vi "VisualizeNiDaqMx.vi"() -> ()   [LabVIEW 2018, in "Visualization.lvlib" / "VisualizeDigitizer.lvclass"]
doc: "This VI listens for any measurement data associated with the provided PluginName and displays it to the user for analysis. The display is only suitable for data coming from the RoomAlert Plugin."
uses:
  VisualizeDigitizer.lvclass
  <vilib>/event_ctls.llb/usereventprio.ctl
  VisualizeBase/VisualizeBase_class/Requests/clUserEventType.ctl
  SubVI/VisulaizationManagement/PopInOutButton.ctl
  <extravilib>/ChannelInstances/Tag-bool/Write With Abort.vi
  <extravilib>/ChannelInstances/Tag-bool/Read With Abort.vi
  <extravilib>/ChannelInstances/Tag-bool/Instantiate.vi
  <extravilib>/ChannelInstances/Tag-bool/EndpointRead.vi
  <vilib>/Utility/error.llb/Error Cluster From Error Code.vi
  <extravilib>/ChannelInstances/Tag-bool/Endpoint.vi
  <vilib>/ErrorRing/Error Ring.xnode
  <userlib>/NIST/NISTErrorLib/NISTErrorLib.lvlib
  VisualizeBase/VisualizeBase_class/VisualizeBase.lvclass
  <extravilib>/ChannelInstances/Tag-bool.lvlib
  TestClass/Test.lvclass
  Queue/Queue.lvlib
  Digitizer/DigitizerModule/DigitizerModule.lvlib
panel:
  in  "ModuleID":i32
  in  "Log Data":bool
  in  "btnStop":bool
  in  "btnReset":bool
  in  "btnClearTest":bool
  out "Siemens":waveform(dbl)[](graph)=[{"t0"=timestamp(3657200531.6397257 s since 1904-01-01), "dt"=1.0, "Y"=[46.19]}, {"t0"=timestamp(3657200531.6397257 s since 1904-01-01), "dt"=1.0, "Y"=[2.0]}, {"t0"=timestamp(3657200531.6397257 s since 1904-01-01), "dt"=1.0, "Y"=[60.0]}]
  out "ErrorArray":errorcluster[](array[cluster])
  in  "PluginName":string="Sensor.RoomAlert1"
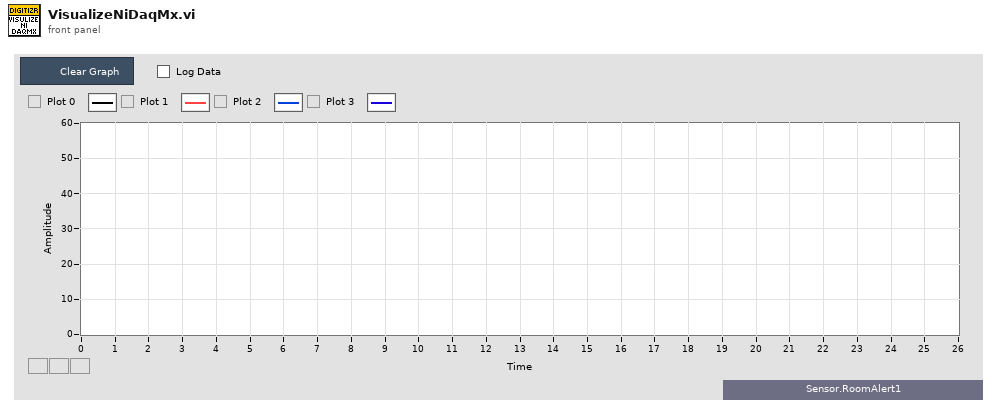
[diagram p1: front panel]
types:
  T1 = enum16{"open", "open or create", "create or replace", "create", "open (read-only)"}
  T2 = typedef "Visualization.lvlib/VisualizeBase.lvclass/clRequestEvents.ctl" = cluster{"StopRequest":refnum<user-event>, "ResetRequest":refnum<user-event>}
  T3 = typedef "DigitizerShared.lvlib/clBroadcastEvents.ctl" = cluster{"DidInit":refnum<user-event>, "StatusUpdate":refnum<user-event>, "ErrorReport":refnum<user-event>, "DidStop":refnum<user-event>, "PathToINI":refnum<user-event>, "Channels":refnum<user-event>, "Acq":refnum<user-event>, "Trigger":refnum<user-event>, "Waveforms":refnum<user-event>}
  T4 = typedef "Visualization.lvlib/VisualizeBase.lvclass/clUserEventType.ctl" = cluster{"BusIndex":i8, "Data":variant}
  T5 = typedef "usereventprio.ctl" = enum32{"high priority", "normal priority"}
  T6 = typedef "Tag-bool.lvlib/))Channel.ctl" = refnum<queue>
  T7 = typedef "PopInOutButton.ctl" = bool
  T8 = typedef "sizeaction.ctl" = enum32{"Minimized", "Maximized", "Resized"}
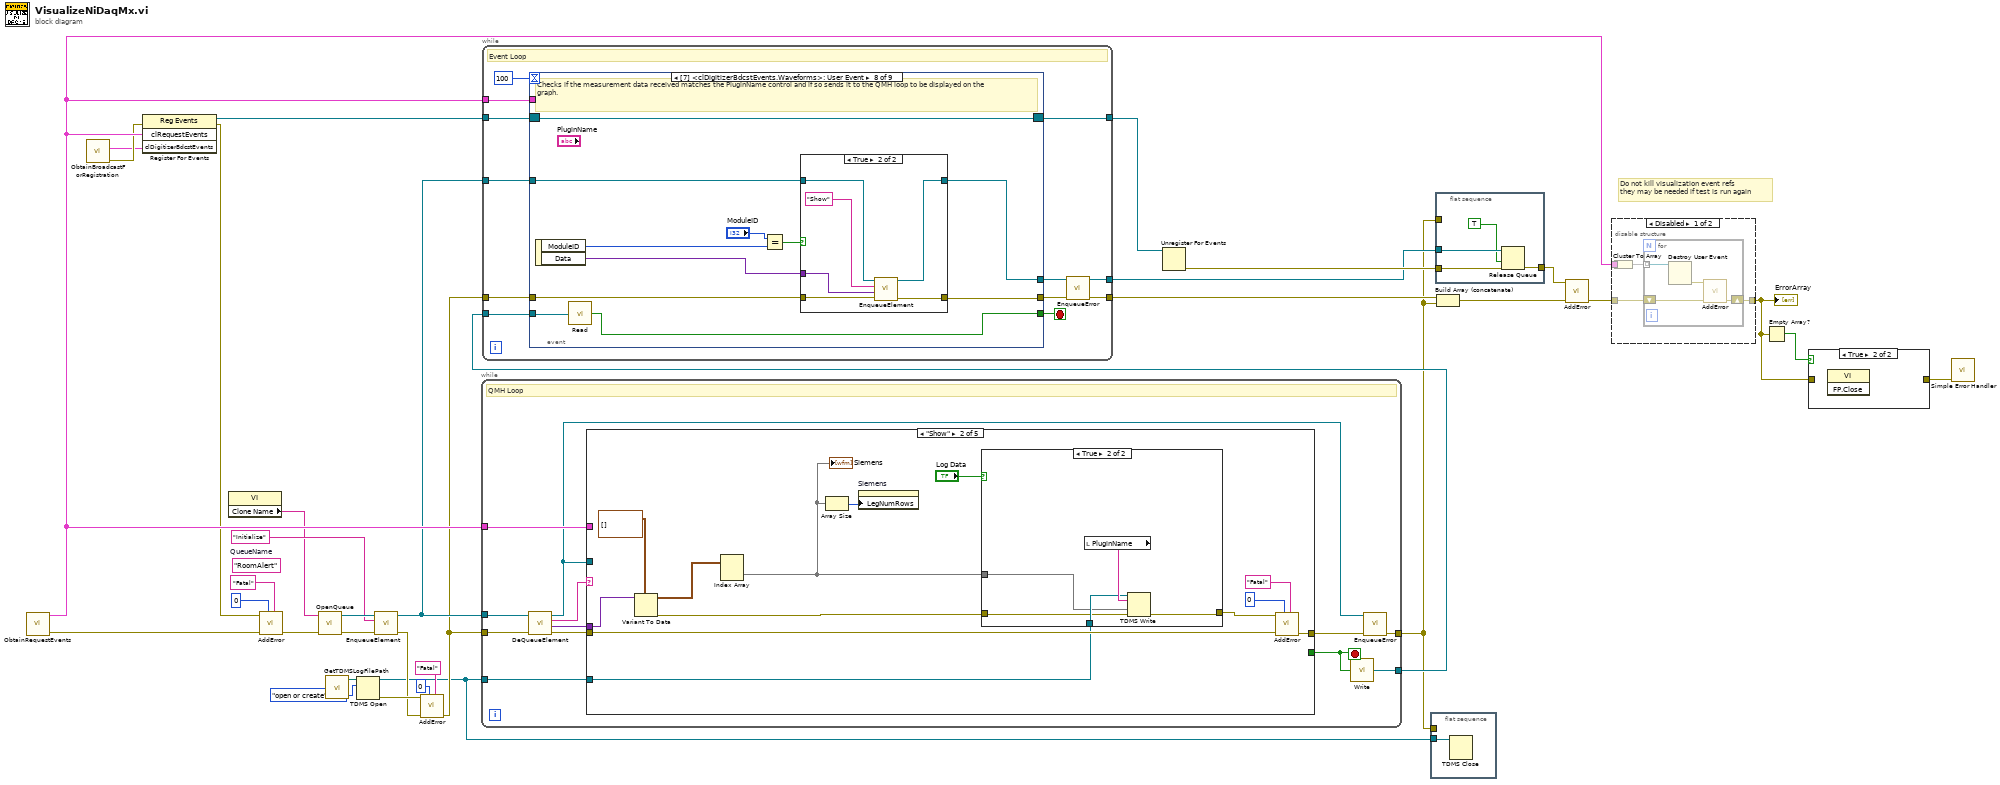
[diagram p0: block diagram]
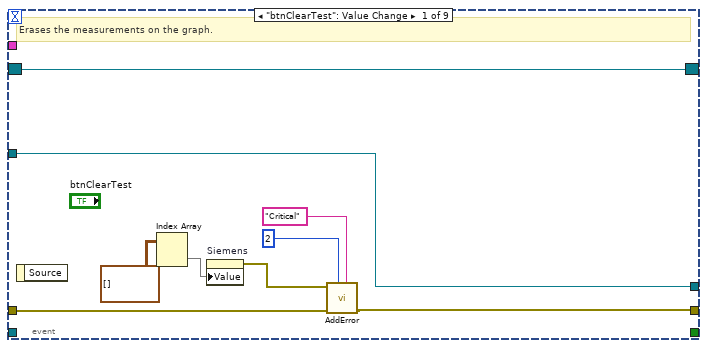
[diagram p3: hidden frame]
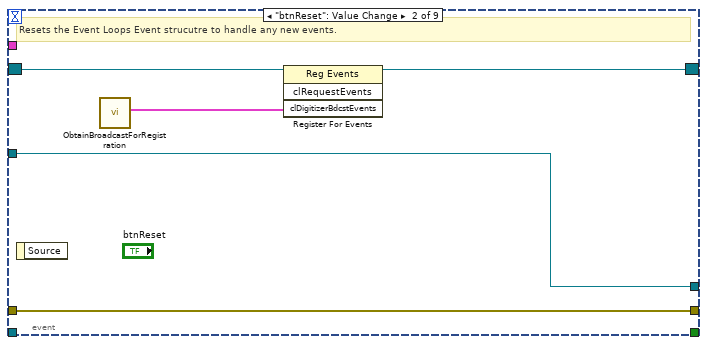
[diagram p4: hidden frame]
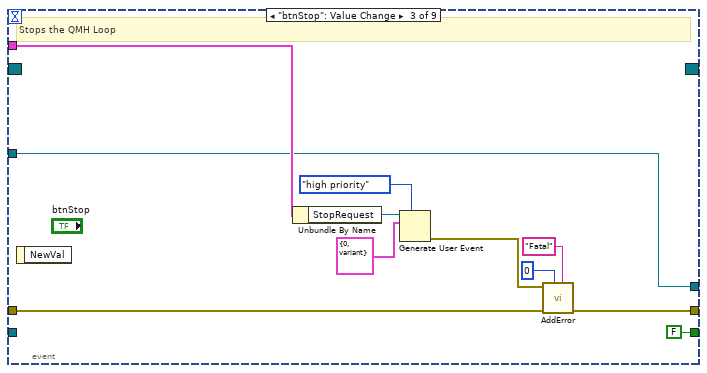
[diagram p5: hidden frame]
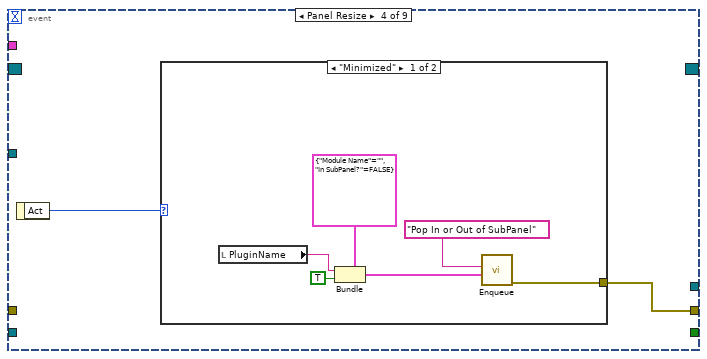
[diagram p6: hidden frame]
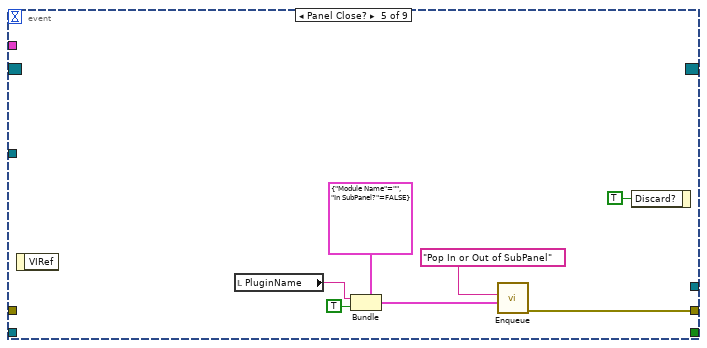
[diagram p8: hidden frame]
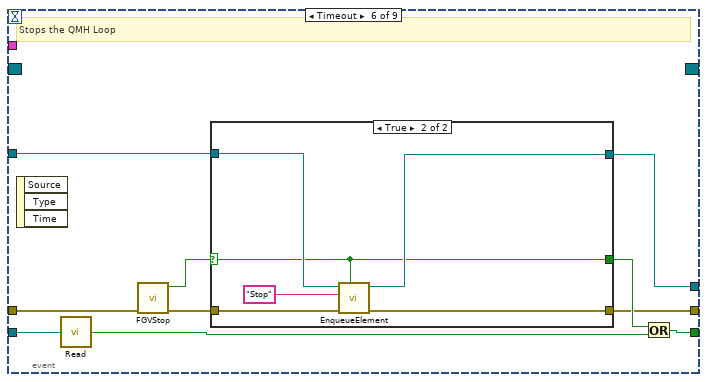
[diagram p9: hidden frame]
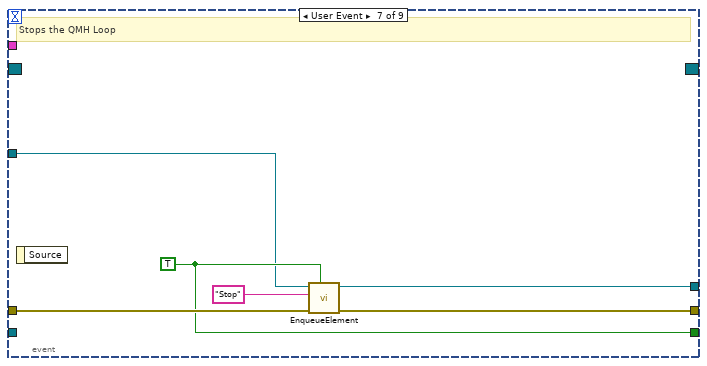
[diagram p11: hidden frame]
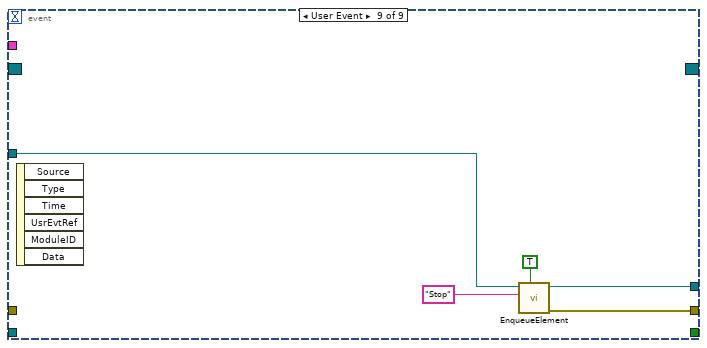
[diagram p13: hidden frame]
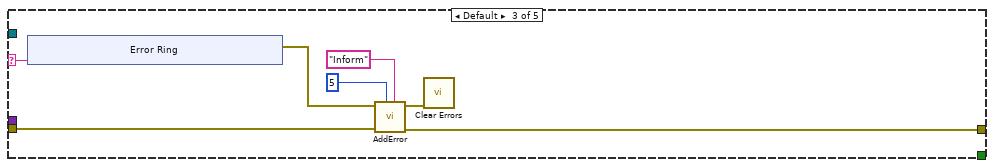
[diagram p16: hidden frame]
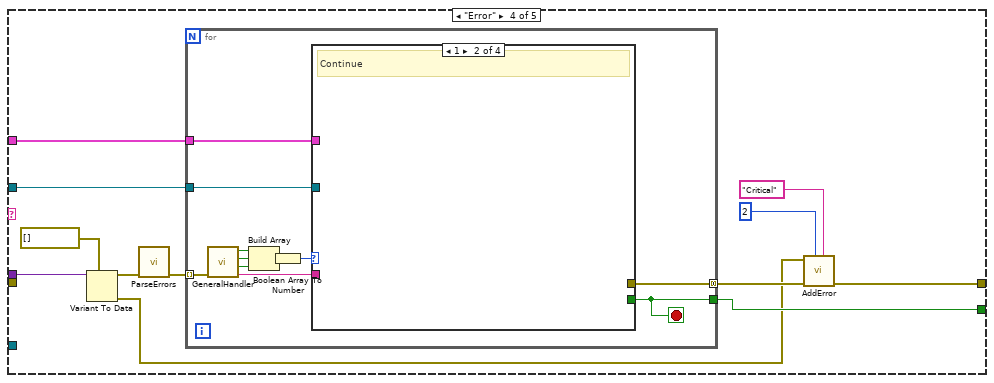
[diagram p17: hidden frame]
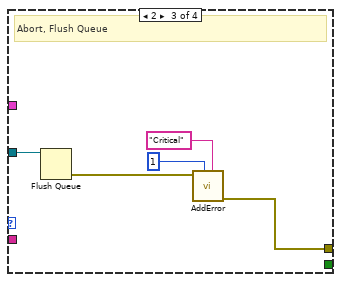
[diagram p19: hidden frame]
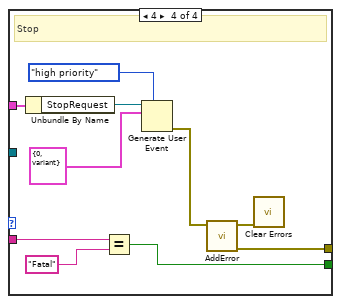
[diagram p20: hidden frame]
diagram:
  (unwired) "RoomAlert"  # QueueName
  # "Do not kill visualization event refs\nthey may be needed if test is run again"
  n1 = call "ObtainRequestEvents.vi"() -> ("Error"=w25:errorcluster[], "clRequestEvents"=w27:T2)  [unwired: 10 in]
  n2 = call "ObtainBroadcastForRegistration.vi"() -> ("error out"=w2:errorcluster, "clDigitizerBdcstEvents"=w1:T3)  [unwired: 10 in]
  n3 = register-events(error in=w2, w27, w1) -> (reference out=w34:refnum<event-registration>, error out=w24:errorcluster)  [unwired: 1 in]
  n4 = property class="VI"() -> ("Clone Name"=w12:string)  [unwired: 2 in, 2 out]
  n5 = call <userlib>:"AddError.vi"("Severity"="Fatal", "Priority"=u8 0, "ErrorArray In"=w25, "error in (no error)"=w24) -> ("ErrorArray Out"=w21:errorcluster[])  [unwired: 6 in, 1 out]
  n6 = call "OpenQueue.vi"("Error Array In"=w21, "QueueName"=w12) -> ("Error Array Out"=w19:errorcluster[], "queue out"=w20:refnum<queue>)  [unwired: 8 in]
  n7 = call "GetTDMSLogFilePath.vi"() -> ("TDMS Log File Path"=w11:path)  [unwired: 11 in]
  n8 = TDMS Open(10:T1."open or create" ("operation (0:open)"), 11:w11) -> (0:w8:errorcluster, 3:w4:refnum<k34>)  [unwired: 5 in]
  n9 = call "EnqueueElement.vi"("Error Array In"=w19, "Message"="Initialize", "queue in"=w20) -> ("Error Array Out"=w7:errorcluster[], "queue out"=w17:refnum<queue>)  [unwired: 7 in]
  n10 = call <userlib>:"AddError.vi"("Severity"="Fatal", "Priority"=u8 0, "ErrorArray In"=w7, "error in (no error)"=w8) -> ("ErrorArray Out"=w6:errorcluster[])  [unwired: 6 in, 1 out]
  n11 = while {
    tunnel: w6 -> [w40]
    tunnel: [w43] -> w3
    tunnel: w17 -> [w39]
    tunnel: w27 -> [w45]
    tunnel: [w36] -> w13
    tunnel: w4 -> [w35]
    stop <- w46 stop-if-true
    # "QMH Loop"
    n12 = call "DeQueueElement.vi"("Error Array In"=w40, "Queue In"=w39) -> ("Error Array Out"=w38:errorcluster[], "Data"=w41:variant, "Message"=w42:string, "Queue Out"=w37:refnum<queue>)  [unwired: 6 in]
    n13 = case shown="\"Show\"" w42 {
      selector: w42 -> [_ _ w73 _ _]
      tunnel: w41 -> [_ w56 _ w92 _]
      tunnel: w38 -> [w47 w59 w71 _ w119]
      tunnel: [w47 w60 w70 w82 w119] -> w44
      tunnel: [_ _ _ w88 TRUE] -> w46
      tunnel: w45 -> [_ _ _ w87 _]
      tunnel: w37 -> [_ _ _ w86 _]
      tunnel: w35 -> [_ w52 _ _ _]
      frame "Initialize" {
      }
      frame "Show" {
        n14 = Variant To Data(type=waveform(dbl)[][] [] ("data"), Variant=w56) -> (data=w49:waveform(dbl)[][], error out=w55:errorcluster)  [unwired: 1 in]
        n15 = Index Array(array=w49) -> (element=w48:waveform(dbl)[])  [unwired: 2 in]
        "Siemens" <- w48
        n16 = Array Size(array=w48) -> (size(s)=w51:i32)
        n17 = property on="Siemens" class="WFGraph (strict)"("LegNumRows"=w51) -> ()  [unwired: 2 in, 2 out]
        n18 = case shown="True" "Log Data" {
          tunnel: w55 -> [w61 w62]
          tunnel: [w61 w66] -> w54
          tunnel: w52 -> [_ w64]
          tunnel: w48 -> [_ w63]
          frame False {
          }
          frame True {
            n19 = local read "PluginName"() -> (w65:string)
            n20 = TDMS Write(0:w64, 5:w65, 9:w63, 11:w62) -> (15:w66:errorcluster)  [unwired: 2 in, 3 out]
          }
        }
        n21 = call <userlib>:"AddError.vi"("Severity"="Fatal" ("String"), "Priority"=u8 0, "ErrorArray In"=w59, "error in (no error)"=w54) -> ("ErrorArray Out"=w60:errorcluster[])  [unwired: 6 in, 1 out]
      }
      frame Default {
        n22 = xnode "Error Ring"("parameter 0"=w73) -> ("error out"=w72:errorcluster)
        n23 = call <userlib>:"AddError.vi"("Severity"="Inform" ("String"), "Priority"=u8 5, "ErrorArray In"=w71, "error in (no error)"=w72) -> ("ErrorArray Out"=w70:errorcluster[], "error out"=w69:errorcluster)  [unwired: 6 in]
        n24 = call <vilib>:"Clear Errors.vi"("error in (no error)"=w69) -> ()  [unwired: 5 in, 2 out]
      }
      frame "Error" {
        n25 = Variant To Data(type=errorcluster[] [], Variant=w92) -> (data=w90:errorcluster[], error out=w81:errorcluster)  [unwired: 1 in]
        n26 = call <userlib>:"ParseErrors.vi"("ErrorArray"=w90) -> ("ErrorArray"=w89:errorcluster[])  [unwired: 8 in, 2 out]
        n27 = for {
          tunnel: w89 -> [w103] mode=indexing
          tunnel: [w97] -> w83 mode=concatenating
          tunnel: [w95] -> w88
          tunnel: w87 -> [w94]
          tunnel: w86 -> [w93]
          stop <- w95 stop-if-true
          n28 = call <userlib>:"GeneralHandler.vi"("error in (no error)"=w103) -> ("Severity"=w96:string, "Stop"=w100:bool, "Abort"=w101:bool, "Continue"=w102:bool)  [unwired: 6 in, 1 out]
          n29 = Build Array(w102, w101, w100) -> (w99:bool[])
          n30 = Boolean Array To Number(Boolean array=w99) -> (number=w98:u32)
          n31 = case shown="1" w98 {
            tunnel: [_ _ w108 w117] -> w97
            tunnel: w96 -> [_ _ _ w110]
            tunnel: [_ _ _ w112] -> w95
            tunnel: w94 -> [_ _ _ w111]
            tunnel: w93 -> [_ _ w104 _]
            frame 0, Default {
              # "No Dialog"
            }
            frame 1 {
              # "Continue"
            }
            frame 2 {
              # "Abort, Flush Queue"
              n32 = Flush Queue(queue=w104) -> (error out=w107:errorcluster)  [unwired: 1 in, 2 out]
              n33 = call <userlib>:"AddError.vi"("Severity"="Critical" ("String"), "Priority"=u8 1, "error in (no error)"=w107) -> ("ErrorArray Out"=w108:errorcluster[])  [unwired: 7 in, 1 out]
            }
            frame 4 {
              # "Stop"
              n34 = Unbundle By Name(w111) -> ("StopRequest"=w118:refnum<user-event>)
              n35 = Equal?(x=w110, y="Fatal" ("x")) -> (x = y?=w112:bool)
              n36 = Generate User Event(priority (normal)=usereventprio."high priority", user event=w118, event data cluster=T4 {"BusIndex"=0, "Data"=variant} ("event data")) -> (error out=w116:errorcluster)  [unwired: 1 in, 1 out]
              n37 = call <userlib>:"AddError.vi"("error in (no error)"=w116) -> ("ErrorArray Out"=w117:errorcluster[], "error out"=w113:errorcluster)  [unwired: 9 in]
              n38 = call <vilib>:"Clear Errors.vi"("error in (no error)"=w113) -> ()  [unwired: 5 in, 2 out]
            }
          }
        }
        n39 = call <userlib>:"AddError.vi"("Severity"="Critical", "Priority"=u8 2, "ErrorArray In"=w83, "error in (no error)"=w81) -> ("ErrorArray Out"=w82:errorcluster[])  [unwired: 6 in, 1 out]
      }
      frame "Stop" {
      }
    }
    n40 = call <extravilib>:"Write.vi"("element"=w46) -> ("channel"=w36:T6)  [unwired: 1 out]
    n41 = call "EnqueueError.vi"("Error Array In"=w44, "Queue in"=w37) -> ("Error Array Out"=w43:errorcluster[])  [unwired: 8 in, 1 out]
  }
  n42 = while {
    tunnel: w34 -> [w132]
    tunnel: [w126] -> w32
    tunnel: [w130] -> w33
    tunnel: w27 -> [w129]
    tunnel: w6 -> [w128]
    tunnel: w17 -> [w127]
    tunnel: [w123] -> w16
    tunnel: w13 -> [w121]
    stop <- w131 stop-if-true
    # "Event Loop"
    n43 = event shown="[7] <clDigitizerBdcstEvents.Waveforms>: User Event" {
      selector: w132 -> [w136 w146 _ _ _ _ _ w204 _]
      dyn-events: [w136 w145 _ _ _ _ _ w204 _] -> w130
      timeout: 100 -> [_ _ _ _ _ _ _ _ _]
      tunnel: [_ _ FALSE ("Priority? (F)") _ _ w173 w194 w201 _] -> w131
      tunnel: [w138 w144 w150 w158 w172 w175 w196 w206 w219] -> w125
      tunnel: w129 -> [_ _ w149 _ _ _ _ _ _]
      tunnel: w128 -> [w139 w144 w157 _ _ w178 w197 w207 _]
      tunnel: w127 -> [w135 w143 w147 _ _ w177 w192 w208 w217]
      tunnel: [w135 w143 w147 _ _ w176 w195 w205 w218] -> w124
      tunnel: w121 -> [_ _ _ _ _ w182 _ w202 _]
      event "btnClearTest": Value Change {
        # "Erases the measurements on the graph."
        n44 = event-data() -> ()  [unwired: 1 in, 1 out]
        n45 = Index Array(array=waveform(dbl)[][] [] ("History Data")) -> (element=w133:waveform(dbl)[])  [unwired: 2 in]
        n46 = property on="Siemens" class="WFGraph (strict)"("Value"=w133) -> (error out=w137:errorcluster)  [unwired: 2 in, 1 out]
        n47 = call <userlib>:"AddError.vi"("Severity"="Critical", "Priority"=u8 2, "ErrorArray In"=w139, "error in (no error)"=w137) -> ("ErrorArray Out"=w138:errorcluster[])  [unwired: 6 in, 1 out]
      }
      event "btnReset": Value Change {
        # "Resets the Event Loops Event strucutre to handle any new events."
        n48 = event-data() -> ()  [unwired: 1 in, 1 out]
        n49 = call "ObtainBroadcastForRegistration.vi"() -> ("clDigitizerBdcstEvents"=w142:T3)  [unwired: 10 in, 1 out]
        n50 = register-events(reference=w146, w142) -> (reference out=w145:refnum<event-registration>)  [unwired: 2 in, 1 out]
      }
      event "btnStop": Value Change {
        # "Stops the QMH Loop"
        n51 = event-data() -> ()  [unwired: 1 in, 1 out]
        n52 = Unbundle By Name(w149) -> ("StopRequest"=w155:refnum<user-event>)
        n53 = Generate User Event(priority (normal)=usereventprio."high priority", user event=w155, event data cluster=T4 {"BusIndex"=0, "Data"=variant} ("event data")) -> (error out=w156:errorcluster)  [unwired: 1 in, 1 out]
        n54 = call <userlib>:"AddError.vi"("Severity"="Fatal" ("String"), "Priority"=u8 0, "ErrorArray In"=w157, "error in (no error)"=w156) -> ("ErrorArray Out"=w150:errorcluster[])  [unwired: 6 in, 1 out]
      }
      event Panel Resize {
        n55 = event-data() -> ("Act"=w159:T8)  [unwired: 1 in]
        n56 = case shown="\"Minimized\"" w159 {
          tunnel: [w160 _] -> w158
          frame "Minimized" {
            n57 = local read "PluginName"() -> (w162:string)
            n58 = Bundle(cluster=cluster{"Module Name":string, "In SubPanel?":T7} {"Module Name"="", "In SubPanel?"=FALSE} ("output cluster"), "Module Name"=w162, "In SubPanel?"=T7 TRUE) -> (w164:cluster{"Module Name":string, "In SubPanel?":T7})
            n59 = call "Enqueue.vi"("Message Data"=w164, "Message"="Pop In or Out of SubPanel") -> ("ErrorArray"=w160:errorcluster[])  [unwired: 9 in]
          }
          frame "Maximized", Default {
          }
        }
      }
      event Panel Close? {
        n60 = event-data() -> ()  [unwired: 1 in, 1 out]
        n61 = local read "PluginName"() -> (w168:string)
        n62 = Bundle(cluster=cluster{"Module Name":string, "In SubPanel?":T7} {"Module Name"="", "In SubPanel?"=FALSE} ("output cluster"), "Module Name"=w168, "In SubPanel?"=T7 TRUE) -> (w170:cluster{"Module Name":string, "In SubPanel?":T7})
        n63 = call "Enqueue.vi"("Message Data"=w170, "Message"="Pop In or Out of SubPanel") -> ("ErrorArray"=w172:errorcluster[])  [unwired: 9 in]
        n64 = event-data("Discard?"=TRUE) -> ()  [unwired: 1 in, 1 out]
      }
      event Timeout {
        # "Stops the QMH Loop"
        n65 = event-data() -> ()  [unwired: 1 in, 3 out]
        n66 = call <extravilib>:"Read.vi"("channel"=w182) -> ("element"=w174:bool)  [unwired: 1 in, 1 out]
        n67 = call "FGVStop.vi"("Error In"=w178) -> ("Error Out"=w180:errorcluster[], "Value"=w181:bool)  [unwired: 9 in]
        n68 = case shown="True" w181 {
          selector: w181 -> [w183 w186]
          tunnel: [w185 w189] -> w175
          tunnel: w180 -> [w185 w190]
          tunnel: w177 -> [w184 w188]
          tunnel: [w184 w187] -> w176
          tunnel: [w183 w186] -> w179
          frame False {
          }
          frame True {
            n69 = call "EnqueueElement.vi"("Priority? (F)"=w186, "Error Array In"=w190, "Message"="Stop", "queue in"=w188) -> ("Error Array Out"=w189:errorcluster[], "queue out"=w187:refnum<queue>)  [unwired: 6 in]
          }
        }
        n70 = Or(x=w179, y=w174) -> (x .or. y?=w173:bool)
      }
      event User Event {
        w194 = TRUE ("Priority? (F)")
        # "Stops the QMH Loop"
        n71 = event-data() -> ()  [unwired: 1 in, 1 out]
        n72 = call "EnqueueElement.vi"("Priority? (F)"=w194, "Error Array In"=w197, "Message"="Stop", "queue in"=w192) -> ("Error Array Out"=w196:errorcluster[], "queue out"=w195:refnum<queue>)  [unwired: 6 in]
      }
      event User Event {
        # "Checks if the measurement data received matches the PluginName control and if so sends it to the QMH loop to be displayed on the graph."
        n73 = event-data() -> ("ModuleID"=w199:i32, "Data"=w200:variant)  [unwired: 1 in]
        n74 = call <extravilib>:"Read.vi"("channel"=w202) -> ("element"=w201:bool)  [unwired: 1 in, 1 out]
        n75 = Equal?(x="ModuleID", y=w199) -> (x = y?=w203:bool)
        n76 = case shown="True" w203 {
          tunnel: [w209 w215] -> w206
          tunnel: w208 -> [w210 w214]
          tunnel: w207 -> [w209 w216]
          tunnel: [w210 w213] -> w205
          tunnel: w200 -> [_ w211]
          frame False {
          }
          frame True {
            n77 = call "EnqueueElement.vi"("Error Array In"=w216, "Data"=w211, "Message"="Show", "queue in"=w214) -> ("Error Array Out"=w215:errorcluster[], "queue out"=w213:refnum<queue>)  [unwired: 6 in]
          }
        }
      }
      event User Event {
        n78 = event-data() -> ()  [unwired: 1 in, 6 out]
        n79 = call "EnqueueElement.vi"("Priority? (F)"=TRUE, "Message"="Stop", "queue in"=w217) -> ("Error Array Out"=w219:errorcluster[], "queue out"=w218:refnum<queue>)  [unwired: 7 in]
      }
    }
    n80 = call "EnqueueError.vi"("Error Array In"=w125, "Queue in"=w124) -> ("Error Array Out"=w126:errorcluster[], "Queue out"=w123:refnum<queue>)  [unwired: 8 in]
  }
  n81 = Unregister For Events(event registration refnum=w33) -> (error out=w31:errorcluster)  [unwired: 1 in]
  n82 = flat-sequence {
    tunnel: w4 -> [w222]
    tunnel: w3 -> [_]
    frame #0 {
      n83 = TDMS Close(11:w222) -> ()  [unwired: 1 in, 2 out]
    }
  }
  n84 = flat-sequence {
    tunnel: w31 -> [w226]
    tunnel: [w225] -> w29
    tunnel: w16 -> [w224]
    tunnel: w3 -> [_]
    frame #0 {
      n85 = Release Queue(queue=w224, force destroy? (F)=TRUE, error in (no error)=w226) -> (error out=w225:errorcluster)  [unwired: 2 out]
    }
  }
  n86 = Build Array (concatenate)(w32, w3) -> (w30:errorcluster[])
  n87 = call <userlib>:"AddError.vi"("ErrorArray In"=w30, "error in (no error)"=w29) -> ("ErrorArray Out"=w28:errorcluster[])  [unwired: 8 in, 1 out]
  n88 = disable-structure shown="Disabled" {
    disable-tunnel: w28 -> [w229 w235]
    disable-tunnel: w27 -> [w228 _]
    disable-tunnel: [w227 w235] -> w15
    frame Disabled {
      n89 = Cluster To Array(cluster=w228) -> (array=w230:refnum<user-event>[])
      n90 = for {
        tunnel: w230 -> [w234] mode=indexing
        shift-right: [w233] -> w227
        shift-left: w229 -> [w232]
        n91 = Destroy User Event(user event=w234) -> (error out=w231:errorcluster)  [unwired: 1 in]
        n92 = call <userlib>:"AddError.vi"("ErrorArray In"=w232, "error in (no error)"=w231) -> ("ErrorArray Out"=w233:errorcluster[])  [unwired: 8 in, 1 out]
      }
    }
    frame Enabled {
    }
  }
  "ErrorArray" <- w15
  n93 = Empty Array?(array=w15) -> (empty?=w26:bool)
  n94 = case shown="True" w26 {
    tunnel: [w236 _] -> w14
    tunnel: w15 -> [w237 _]
    frame False {
      n95 = Merge Errors(w237) -> (w236:errorcluster)
    }
    frame True {
      n96 = invoke class="VI" method="FP.Close"() -> ()  [unwired: 3 in, 3 out]
    }
  }
  n97 = call <vilib>:"Simple Error Handler.vi"("error in (no error)"=w14) -> ()  [unwired: 4 in, 5 out]
